vi "Init.vi"(5 "PathControl.lvclass":refnum<class "PathControl.lvclass">, 6 "Environmental classes":refnum<class "Instrument.lvclass">[](array[class]), 7 "XML Handler.lvclass":refnum<class "XML Handler.lvclass">, 8 "error in (no error)":errorcluster, 9 "Instruments to Use":T1(array[cluster]), 10 "Device.lvclass":refnum<class "Device.lvclass">, 11 "DC in":refnum<class "DC.lvclass">) -> (0 "error out":errorcluster, 3 "DC out":refnum<class "DC.lvclass">)   [LabVIEW 2020, in "DC.lvclass"]
doc: "Initializes the measurement.\nThis verifies that the instruments are present and adds them into the class data.\nIs also adds the xml handler into the class data."
uses:
  DC.lvclass
  Devices/Device.lvclass
  Instruments/Instrument.lvclass
  XML Handler/XML Handler.lvclass
  Path Control/PathControl.lvclass
  Controls/Init State Machine.ctl
  Measurement.lvclass
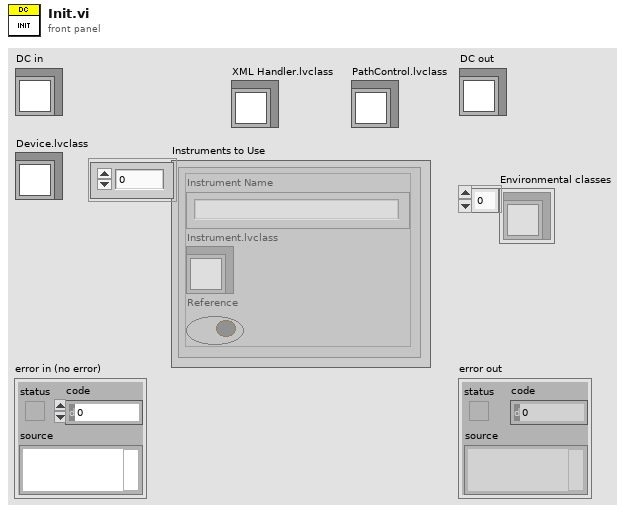
[diagram p1: front panel]
types:
  T1 = cluster{"Instrument Name":string, "Instrument.lvclass":refnum<class "Instrument.lvclass">, "Reference":bool}[]
  T2 = typedef "DC.lvclass/Init State Machine.ctl" = enum16{"Verify Instruments", "Init Instruments", "Done"}
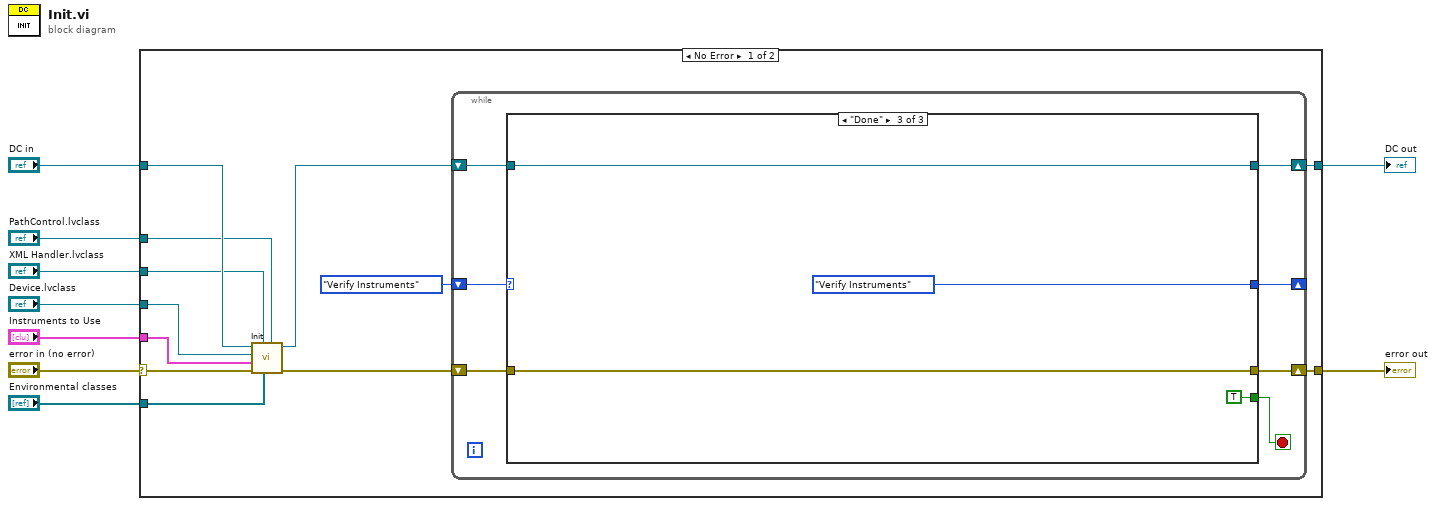
[diagram p0: block diagram]
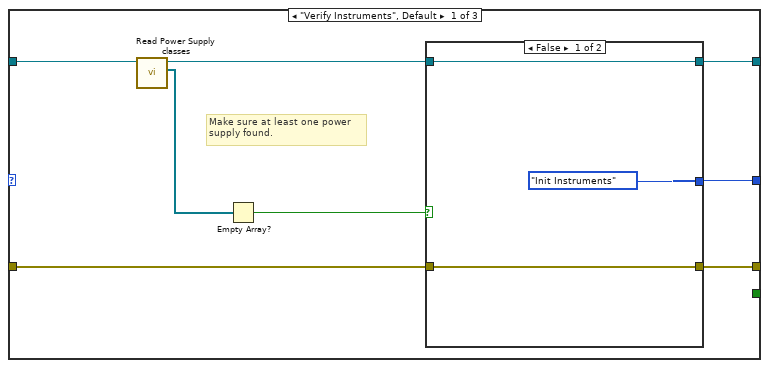
[diagram p2: hidden frame]
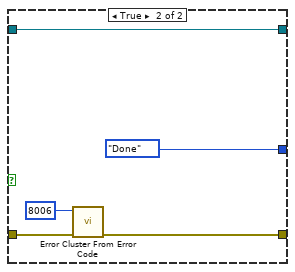
[diagram p3: hidden frame]
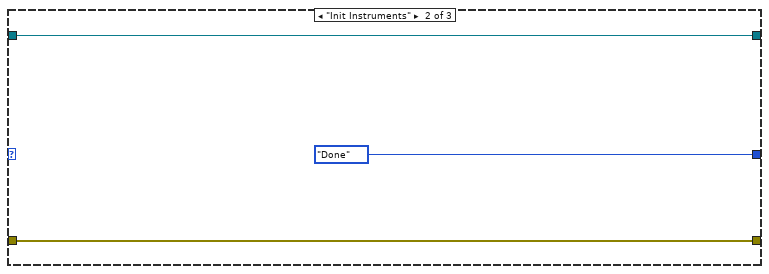
[diagram p4: hidden frame]
diagram:
  n1 = case shown="No Error" "error in (no error)" {
    selector: "error in (no error)" -> [w19 w52]
    tunnel: "DC in" -> [w17 w53]
    tunnel: "Instruments to Use" -> [w11 _]
    tunnel: [w21 w53] -> w6
    tunnel: [w20 w52] -> w5
    tunnel: "Device.lvclass" -> [w14 _]
    tunnel: "XML Handler.lvclass" -> [w13 _]
    tunnel: "PathControl.lvclass" -> [w12 _]
    tunnel: "Environmental classes" -> [w10 _]
    frame No Error {
      n2 = call-parent "Init.vi"("PathControl.lvclass"=w12, "Environmental classes"=w10, "XML Handler.lvclass"=w13, "error in (no error)"=w19, "Instruments to Use"=w11, "Device.lvclass"=w14, "Measurements in"=w17) -> ("error out"=w18:errorcluster, "Measurements out"=w16:refnum<class "DC.lvclass">)  [unwired: 3 in]
      n3 = while {
        shift-right: [w27] -> w21
        shift-left: w16 -> [w28]
        shift-right: [w25] -> _
        shift-left: Init_State_Machine."Verify Instruments" -> [w26]
        shift-right: [w23] -> w20
        shift-left: w18 -> [w24]
        stop <- w22 stop-if-true
        n4 = case shown="\"Done\"" w26 {
          tunnel: w28 -> [w32 w47 w51]
          tunnel: [w36 w47 w51] -> w27
          tunnel: [w33 Init_State_Machine."Done" Init_State_Machine."Verify Instruments"] -> w25
          tunnel: w24 -> [w35 w46 w50]
          tunnel: [w34 w46 w50] -> w23
          tunnel: [_ _ TRUE] -> w22
          frame "Verify Instruments", Default {
            # "Make sure at least one power \nsupply found."
            n5 = call-dynamic "Read Power Supply classes.vi"("Measurements in"=w32) -> ("Power Supply classes"=w30:refnum<class "Power Supply.lvclass">[], "Measurements out"=w31:refnum<class "DC.lvclass">)  [unwired: 9 in]
            n6 = Empty Array?(array=w30) -> (empty?=w29:bool)
            n7 = case shown="False" w29 {
              tunnel: w31 -> [w39 w44]
              tunnel: [w39 w44] -> w36
              tunnel: w35 -> [w38 w43]
              tunnel: [w38 w41] -> w34
              tunnel: [Init_State_Machine."Init Instruments" Init_State_Machine."Done"] -> w33
              frame False {
              }
              frame True {
                n8 = call <vilib>:"Error Cluster From Error Code.vi"("error in (no error)"=w43, "error code (0)"=8006) -> ("error out"=w41:errorcluster)  [unwired: 7 in]
              }
            }
          }
          frame "Init Instruments" {
          }
          frame "Done" {
          }
        }
      }
    }
    frame Error {
    }
  }
  "error out" <- w5
  "DC out" <- w6
